vi "PI_CheckScan.vi"(0 "Picture size":dbl min=0.1 max=200.0 format="%1.1f um", 1 "Picture size 2":dbl min=0.1 max=200.0 format="%1.1f um", 2 "Axis":enum32{"x-y", "x-z", "y-x", "y-z", "z-x", "z-y"}(ring), 3 "x-Position":dbl, 4 "y-Position":dbl, 5 "z-Position":dbl, 7 "error in (no error)":errorcluster caption="Fehler (Eingang, kein Fehler)") -> (13 "error out":errorcluster caption="Fehler (Ausgang)", 14 "Picture size out":dbl min=0.1 max=200.0 format="%1.1f um", 15 "Picture size out 2":dbl min=0.1 max=200.0 format="%1.1f um", 17 "a0":dbl, 18 "b0":dbl, 19 "c0":dbl)   [LabVIEW 2009]
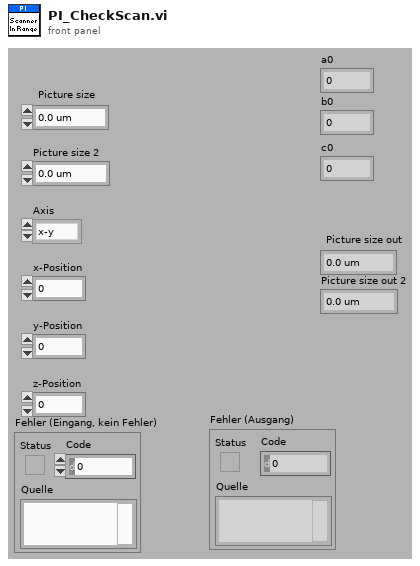
[diagram p1: front panel]
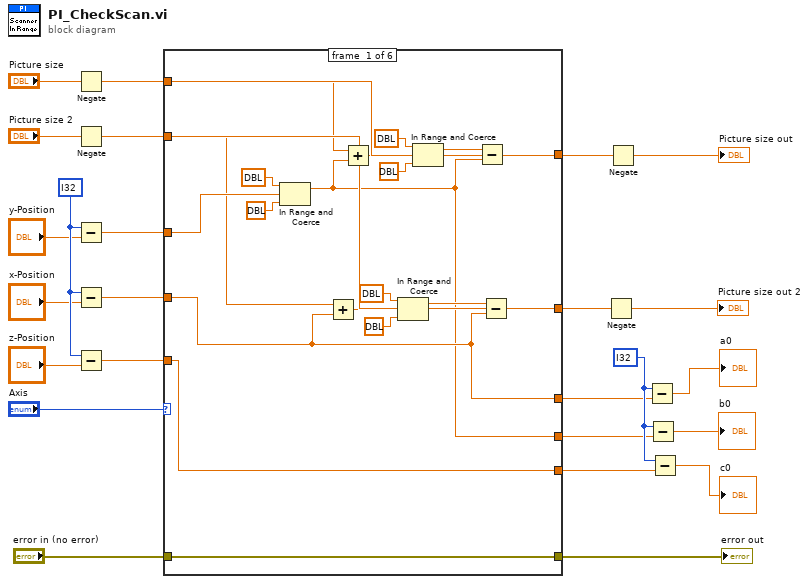
[diagram p0: block diagram]
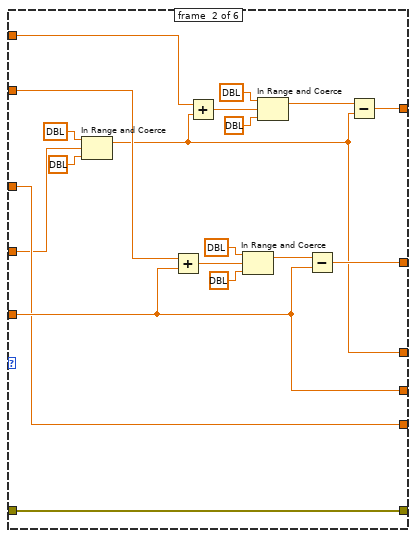
[diagram p2: hidden frame]
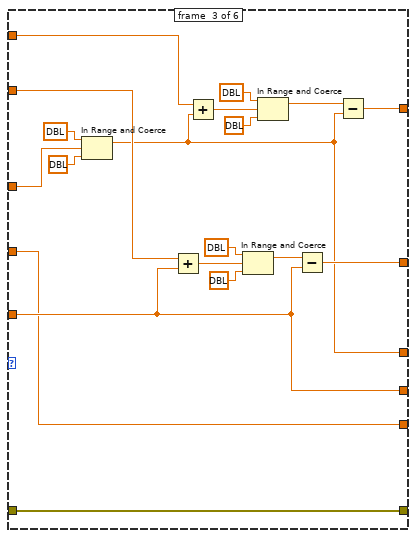
[diagram p3: hidden frame]
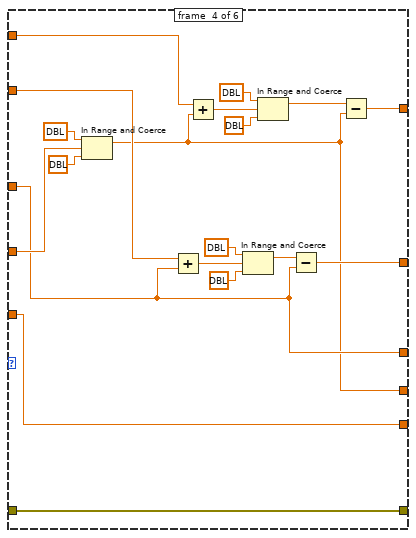
[diagram p4: hidden frame]
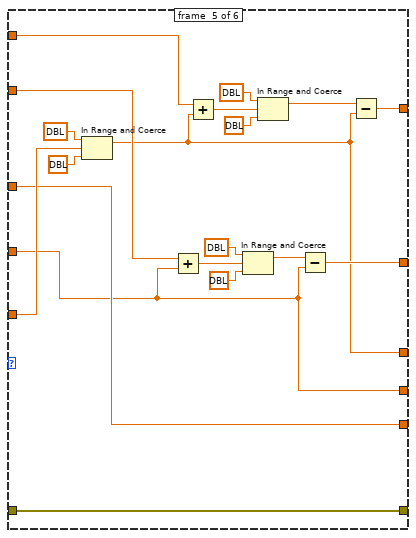
[diagram p5: hidden frame]
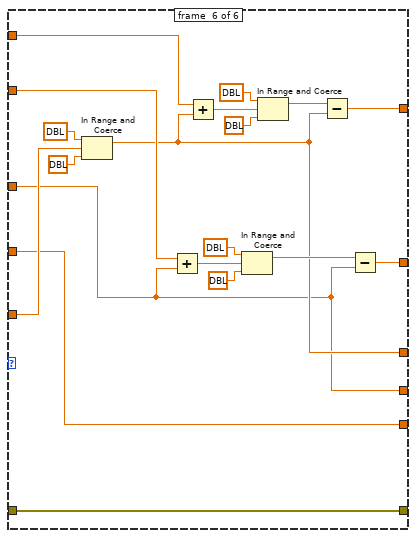
[diagram p6: hidden frame]
diagram:
  w8 = i32 ?
  w16 = i32 ?
  n1 = Negate(x="Picture size") -> (-x=w15:dbl)
  n2 = Negate(x="Picture size 2") -> (-x=w14:dbl)
  n3 = Subtract(x=w16, y="y-Position") -> (x-y=w19:dbl)
  n4 = Subtract(x=w16, y="x-Position") -> (x-y=w18:dbl)
  n5 = Subtract(x=w16, y="z-Position") -> (x-y=w17:dbl)
  n6 = case shown="\"z-y\"" "Axis" {
    tunnel: w15 -> [w29 w49 w68 w87 w106 w125]
    tunnel: w14 -> [w27 w48 w67 w86 w105 w124]
    tunnel: w18 -> [w25 w43 w62 w85 w100 w120]
    tunnel: w19 -> [w30 w44 w63 w82 w101 w119]
    tunnel: w17 -> [w28 w46 w66 w84 w104 w123]
    tunnel: [w34 w53 w72 w91 w110 w129] -> _
    tunnel: [w33 w52 w71 w90 w109 w128] -> _
    tunnel: [w28 w44 w62 w84 w101 w120] -> w7
    tunnel: [w24 w46 w66 w81 w100 w119] -> w6
    tunnel: [w25 w47 w65 w82 w103 w122] -> w5
    tunnel: "error in (no error)" -> [w26 w45 w64 w83 w102 w121]
    tunnel: [w26 w45 w64 w83 w102 w121] -> w3
    frame #0 {
      n7 = In Range and Coerce(upper limit=dbl ?, x=w30, lower limit=dbl ?) -> (coerced(x)=w24:dbl)  [unwired: 1 out]
      n8 = Add(x=w27, y=w25) -> (x+y=w41:dbl)
      n9 = Add(x=w29, y=w24) -> (x+y=w42:dbl)
      n10 = In Range and Coerce(upper limit=dbl ?, x=w41, lower limit=dbl ?) -> (coerced(x)=w35:dbl)  [unwired: 1 out]
      n11 = In Range and Coerce(upper limit=dbl ?, x=w42, lower limit=dbl ?) -> (coerced(x)=w36:dbl)  [unwired: 1 out]
      n12 = Subtract(x=w36, y=w24) -> (x-y=w34:dbl)
      n13 = Subtract(x=w35, y=w25) -> (x-y=w33:dbl)
    }
    frame #1 {
      n14 = In Range and Coerce(upper limit=dbl ?, x=w43, lower limit=dbl ?) -> (coerced(x)=w47:dbl)  [unwired: 1 out]
      n15 = Add(x=w48, y=w46) -> (x+y=w60:dbl)
      n16 = Add(x=w49, y=w47) -> (x+y=w61:dbl)
      n17 = In Range and Coerce(upper limit=dbl ?, x=w60, lower limit=dbl ?) -> (coerced(x)=w54:dbl)  [unwired: 1 out]
      n18 = In Range and Coerce(upper limit=dbl ?, x=w61, lower limit=dbl ?) -> (coerced(x)=w55:dbl)  [unwired: 1 out]
      n19 = Subtract(x=w54, y=w46) -> (x-y=w52:dbl)
      n20 = Subtract(x=w55, y=w47) -> (x-y=w53:dbl)
    }
    frame #2 {
      n21 = In Range and Coerce(upper limit=dbl ?, x=w63, lower limit=dbl ?) -> (coerced(x)=w65:dbl)  [unwired: 1 out]
      n22 = Add(x=w67, y=w66) -> (x+y=w79:dbl)
      n23 = Add(x=w68, y=w65) -> (x+y=w80:dbl)
      n24 = In Range and Coerce(upper limit=dbl ?, x=w79, lower limit=dbl ?) -> (coerced(x)=w73:dbl)  [unwired: 1 out]
      n25 = In Range and Coerce(upper limit=dbl ?, x=w80, lower limit=dbl ?) -> (coerced(x)=w74:dbl)  [unwired: 1 out]
      n26 = Subtract(x=w73, y=w66) -> (x-y=w71:dbl)
      n27 = Subtract(x=w74, y=w65) -> (x-y=w72:dbl)
    }
    frame #3 {
      n28 = In Range and Coerce(upper limit=dbl ?, x=w85, lower limit=dbl ?) -> (coerced(x)=w81:dbl)  [unwired: 1 out]
      n29 = Add(x=w86, y=w82) -> (x+y=w98:dbl)
      n30 = Add(x=w87, y=w81) -> (x+y=w99:dbl)
      n31 = In Range and Coerce(upper limit=dbl ?, x=w98, lower limit=dbl ?) -> (coerced(x)=w92:dbl)  [unwired: 1 out]
      n32 = In Range and Coerce(upper limit=dbl ?, x=w99, lower limit=dbl ?) -> (coerced(x)=w93:dbl)  [unwired: 1 out]
      n33 = Subtract(x=w92, y=w82) -> (x-y=w90:dbl)
      n34 = Subtract(x=w93, y=w81) -> (x-y=w91:dbl)
    }
    frame #4 {
      n35 = In Range and Coerce(upper limit=dbl ?, x=w104, lower limit=dbl ?) -> (coerced(x)=w103:dbl)  [unwired: 1 out]
      n36 = Add(x=w105, y=w100) -> (x+y=w117:dbl)
      n37 = Add(x=w106, y=w103) -> (x+y=w118:dbl)
      n38 = In Range and Coerce(upper limit=dbl ?, x=w117, lower limit=dbl ?) -> (coerced(x)=w111:dbl)  [unwired: 1 out]
      n39 = In Range and Coerce(upper limit=dbl ?, x=w118, lower limit=dbl ?) -> (coerced(x)=w112:dbl)  [unwired: 1 out]
      n40 = Subtract(x=w111, y=w100) -> (x-y=w109:dbl)
      n41 = Subtract(x=w112, y=w103) -> (x-y=w110:dbl)
    }
    frame #5 {
      n42 = In Range and Coerce(upper limit=dbl ?, x=w123, lower limit=dbl ?) -> (coerced(x)=w122:dbl)  [unwired: 1 out]
      n43 = Add(x=w124, y=w119) -> (x+y=w136:dbl)
      n44 = Add(x=w125, y=w122) -> (x+y=w137:dbl)
      n45 = In Range and Coerce(upper limit=dbl ?, x=w136, lower limit=dbl ?) -> (coerced(x)=w130:dbl)  [unwired: 1 out]
      n46 = In Range and Coerce(upper limit=dbl ?, x=w137, lower limit=dbl ?) -> (coerced(x)=w131:dbl)  [unwired: 1 out]
      n47 = Subtract(x=w131, y=w122) -> (x-y=w129:dbl)
      n48 = Subtract(x=w130, y=w119) -> (x-y=w128:dbl)
    }
  }
  "error out" <- w3
  n49 = Negate(x=w14) -> (-x=→"Picture size out 2":dbl)
  n50 = Negate(x=w15) -> (-x=→"Picture size out":dbl)
  n51 = Subtract(x=w8, y=w5) -> (x-y=→"a0":dbl)
  n52 = Subtract(x=w8, y=w6) -> (x-y=→"b0":dbl)
  n53 = Subtract(x=w8, y=w7) -> (x-y=→"c0":dbl)
